vi "Initialize-UI-and-storage-buffer-refs.vi"(8 "error in (no error)":errorcluster, 9 "Number of cameras":i32, 10 "Batch size":i32, 11 "Buffers in":refnum<class "CV-Buffers.lvclass">) -> (0 "error out":errorcluster, 3 "Buffers out":refnum<class "CV-Buffers.lvclass">)   [LabVIEW 2013, in "CameraVision.lvlib" / "CV-Buffers.lvclass"]
uses:
  CV-Buffers.lvclass
  Storage-buffer-refs.ctl
  <vilib>/vision/Image Controls.llb/IMAQ Image.ctl
  CV-Buffers.lvclass/CV-Buffers.ctl
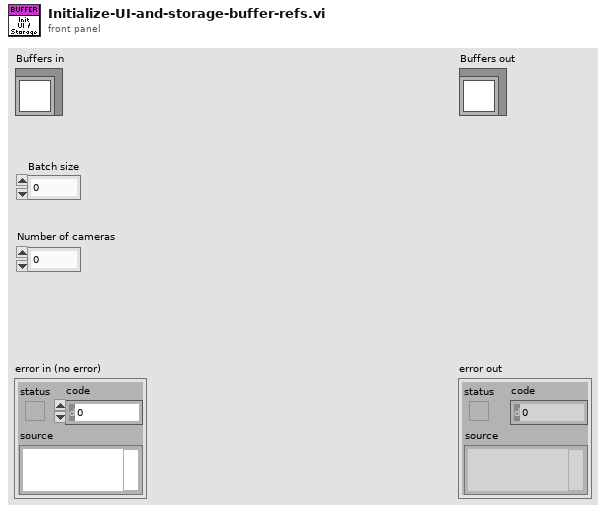
[diagram p1: front panel]
types:
  T1 = typedef "CameraVision.lvlib/CV-Buffers.lvclass/Storage-buffer-refs.ctl" = cluster{"Raw images":T2[], "Corrected images":T2[], "Binary images":T2[]}
  T2 = typedef "IMAQ Image.ctl" = refnum<image>
  T3 = typedef "Image Type" = u32
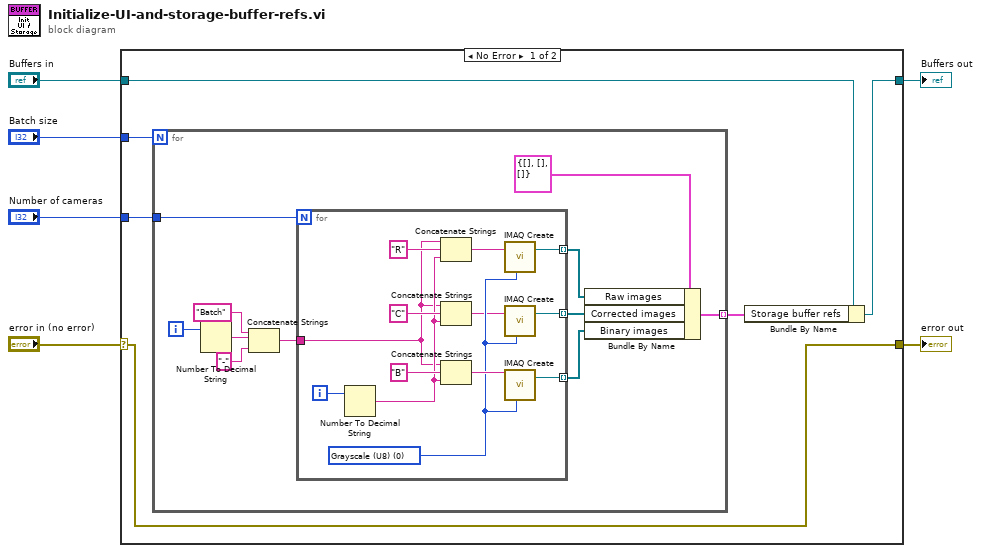
[diagram p0: block diagram]
diagram:
  n1 = case shown="No Error" "error in (no error)" {
    selector: "error in (no error)" -> [w11 w38]
    tunnel: [w11 w38] -> w5
    tunnel: [w8 w37] -> w3
    tunnel: "Buffers in" -> [w12 w37]
    tunnel: "Batch size" -> [w10 _]
    tunnel: "Number of cameras" -> [w9 _]
    frame No Error {
      n2 = for {
        N: w10 -> [_]
        tunnel: [w14] -> w7 mode=indexing
        tunnel: w9 -> [w13]
        i -> [w23]
        n3 = Number To Decimal String(number=w23) -> (decimal integer string=w22:string)  [unwired: 1 in]
        n4 = Concatenate Strings("Batch" ("string"), w22, "-" ("string")) -> (w19:string)
        n5 = for {
          N: w13 -> [_]
          tunnel: w19 -> [w26]
          tunnel: [w34] -> w15 mode=indexing
          tunnel: [w32] -> w17 mode=indexing
          tunnel: [w30] -> w16 mode=indexing
          i -> [w36]
          w31 = T3 0 items=["Grayscale (U8)", "Grayscale (I16)", "Grayscale (SGL)", "Complex (CSG)", "RGB (U32)", "HSL (U32)", "RGB (U64)", "Grayscale (U16)"] ("Image Type")
          n6 = Number To Decimal String(number=w36) -> (decimal integer string=w27:string)  [unwired: 1 in]
          n7 = Concatenate Strings(w26, "R" ("string"), w27) -> (w25:string)
          n8 = Concatenate Strings(w26, "C" ("string"), w27) -> (w24:string)
          n9 = Concatenate Strings(w26, "B" ("string"), w27) -> (w35:string)
          n10 = call "IMAQ Create"("Image Name"=w25, "Image Type"=w31) -> ("New Image"=w30:T2)  [unwired: 3 in, 1 out]
          n11 = call "IMAQ Create"("Image Name"=w24, "Image Type"=w31) -> ("New Image"=w32:T2)  [unwired: 3 in, 1 out]
          n12 = call "IMAQ Create"("Image Name"=w35, "Image Type"=w31) -> ("New Image"=w34:T2)  [unwired: 3 in, 1 out]
        }
        n13 = Bundle By Name(cluster=T1 {"Raw images"=[], "Corrected images"=[], "Binary images"=[]} ("Storage element"), "Raw images"=w16, "Corrected images"=w17, "Binary images"=w15) -> (w14:T1)
      }
      n14 = Bundle By Name(cluster=w12, "Storage buffer refs"=w7) -> (w8:refnum<class "CV-Buffers.lvclass">)
    }
    frame Error {
    }
  }
  "error out" <- w5
  "Buffers out" <- w3
